vi "Open RFSA.vi"(8 "error in":errorcluster {"code" format="%.0x"}, 10 "Bitfile":string="niVSTFPGA_UART.lvbitx", 11 "resource name":refnum<k15>) -> (0 "error out":errorcluster {"code" format="%.0x"}, 3 "instrument handle out":refnum<k15>)   [LabVIEW 2018]
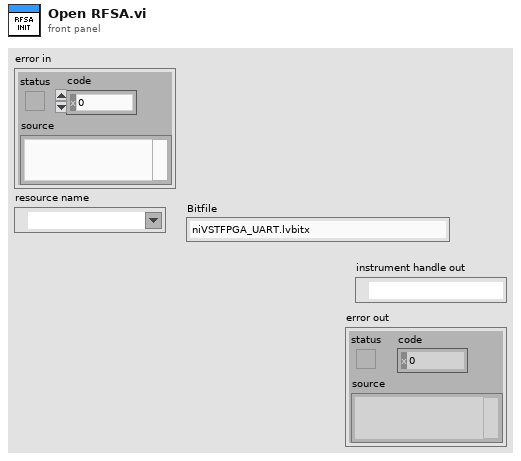
[diagram p1: front panel]
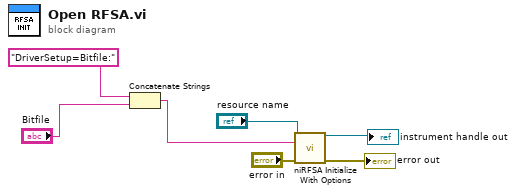
[diagram p0: block diagram]
diagram:
  n1 = Concatenate Strings("DriverSetup=Bitfile:" ("string"), "Bitfile") -> (w5:string)
  n2 = call <instrlib>:"niRFSA Initialize With Options.vi"("resource name"="resource name", "option string"=w5, "error in"="error in") -> ("instrument handle out"=→"instrument handle out":refnum<k15>, "error out"=→"error out":errorcluster)  [unwired: 11 in]
